vi "FTW-Ether-Address-Build.vi"(5 "Path":string, 7 "Message Transport Scheme":T2, 11 "error in":errorcluster) -> (6 "Endpoint Address":T1, 15 "error out":errorcluster)   [LabVIEW 2012, in "FTW-Actor.lvlib" / "FTW-Ether.lvclass"]
uses:
  FTW-Ether.lvclass
  FTW-Ether-MessageTransportScheme.ctl
  Utility/FTW-Actor-Address.ctl
  FTW-Actor.lvlib
panel:
  # "Inputs"
  # "Outputs"
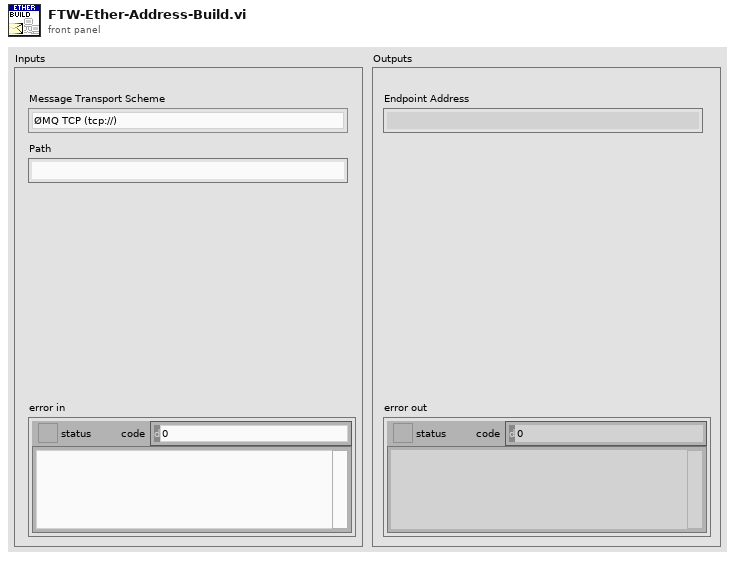
[diagram p1: front panel]
types:
  T1 = typedef "FTW-Actor.lvlib/FTW-Actor-Address.ctl" = string
  T2 = typedef "FTW-Actor.lvlib/FTW-Ether.lvclass/FTW-Ether-MessageTransportScheme.ctl" = enum16{"ØMQ TCP (tcp://)", "ØMQ In-Process (inproc://)", "LabVIEW Queues (lvq://)", "LabVIEW Network Streams (lvns://)"}
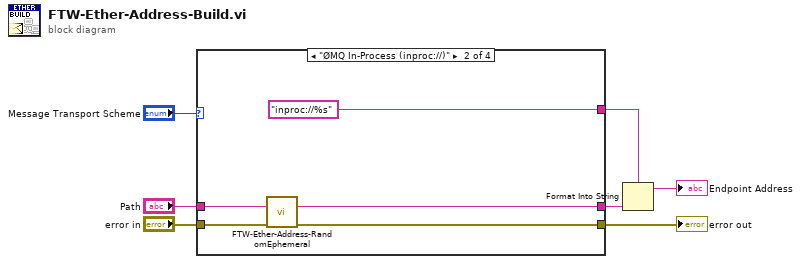
[diagram p0: block diagram]
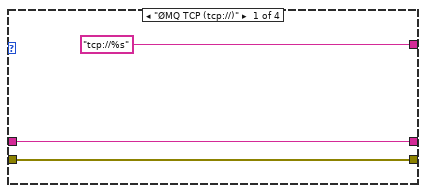
[diagram p2: hidden frame]
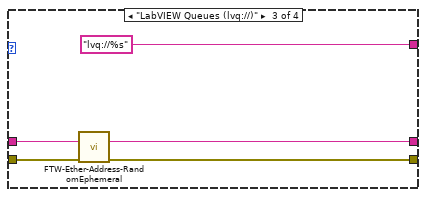
[diagram p3: hidden frame]
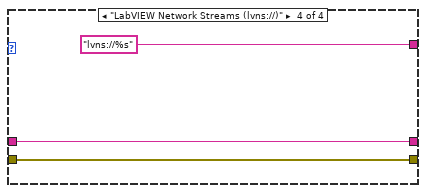
[diagram p4: hidden frame]
diagram:
  n1 = case shown="\"ØMQ In-Process (inproc://)\"" "Message Transport Scheme" {
    tunnel: ["tcp://%s" ("format string") "inproc://%s" ("format string") "lvq://%s" ("format string") "lvns://%s" ("format string")] -> w6
    tunnel: "Path" -> [w9 w14 w19 w22]
    tunnel: [w9 w12 w16 w22] -> w3
    tunnel: "error in" -> [w8 w13 w18 w21]
    tunnel: [w8 w11 w17 w21] -> w1
    frame "ØMQ TCP (tcp://)" {
    }
    frame "ØMQ In-Process (inproc://)" {
      n2 = call "FTW-Ether-Address-RandomEphemeral.vi"("Endpoint"=w14, "error in"=w13) -> ("Endpoint with Replacements"=w12:T1, "error out"=w11:errorcluster)  [unwired: 12 in]
    }
    frame "LabVIEW Queues (lvq://)" {
      n3 = call "FTW-Ether-Address-RandomEphemeral.vi"("Endpoint"=w19, "error in"=w18) -> ("Endpoint with Replacements"=w16:T1, "error out"=w17:errorcluster)  [unwired: 12 in]
    }
    frame "LabVIEW Network Streams (lvns://)" {
    }
  }
  "error out" <- w1
  n4 = Format Into String(format string=w6, w3) -> (resulting string=→"Endpoint Address":string)  [unwired: 2 in, 1 out]
